vi "SetFPLocn.vi"(10 "Cluster":T1) -> (0 "error out":errorcluster)   [LabVIEW 2021]
uses:
  Anemometry Sub Vis/Controls/VInameSizePath.ctl
  <vilib>/Utility/miscctls.llb/LVRectTypeDef.ctl
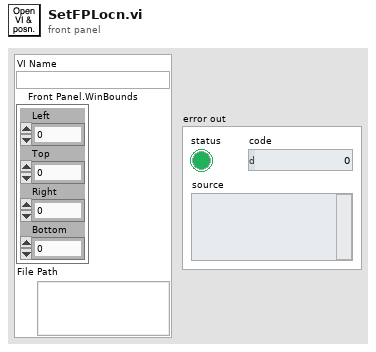
[diagram p1: front panel]
types:
  T1 = typedef "VInameSizePath.ctl" = cluster{"VI Name":string, "Front Panel.WinBounds":T2, "File Path":path}
  T2 = typedef "LVRectTypeDef.ctl" = cluster{"Left":i16, "Top":i16, "Right":i16, "Bottom":i16}
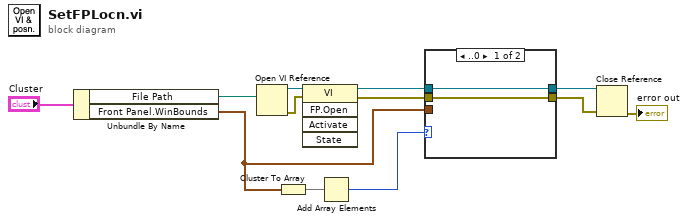
[diagram p0: block diagram]
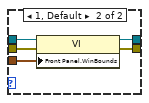
[diagram p2: hidden frame]
diagram:
  n1 = Unbundle By Name("Cluster") -> ("File Path"=w9:path, "Front Panel.WinBounds"=w3:T2)
  n2 = Open VI Reference(vi path=w9) -> (vi reference=w12:refnum<vi>, error out=w7:errorcluster)  [unwired: 5 in]
  n3 = Cluster To Array(cluster=w3) -> (array=w2:i16[])
  n4 = invoke class="VI" method="FP.Open"(reference=w12, error in=w7) -> (reference out=w8:refnum<vi>, error out=w6:errorcluster)  [unwired: 3 in, 3 out]
  n5 = Add Array Elements(numeric array=w2) -> (sum=w1:i16)
  n6 = case shown="..0" w1 {
    tunnel: [w14 w19] -> w11
    tunnel: w8 -> [w14 w18]
    tunnel: w6 -> [w13 w17]
    tunnel: [w13 w16] -> w5
    tunnel: w3 -> [_ w15]
    frame ..0 {
    }
    frame 1, Default {
      n7 = property class="VI"(reference=w18, error in=w17, "Front Panel.WinBounds"=w15) -> (reference out=w19:refnum<vi>, error out=w16:errorcluster)
    }
  }
  n8 = Close Reference(reference=w11, error in (no error)=w5) -> (error out=→"error out":errorcluster)
